vi "Configure Time Domain Reflection Type.vi"(7 "Cable Loss Value (0)":dbl, 8 "error in (no error)":errorcluster, 9 "Reflection Type (1: Round Trip)":i32(ring)=1 items=["One Way", "Round Trip"], 10 "Channel (1)":i32=1, 11 "VISA resource name":refnum<visa-resource-name>) -> (0 "error out":errorcluster, 3 "VISA resource name out":refnum<visa-resource-name>)   [LabVIEW 2011, in "Agilent ENA Series.lvlib"]
doc: "This VI configures time domain reflection type and cable loss value.\n\n<B>Note:</B>This VI is only vaild on E5061B."
uses:
  Agilent ENA Series.lvlib
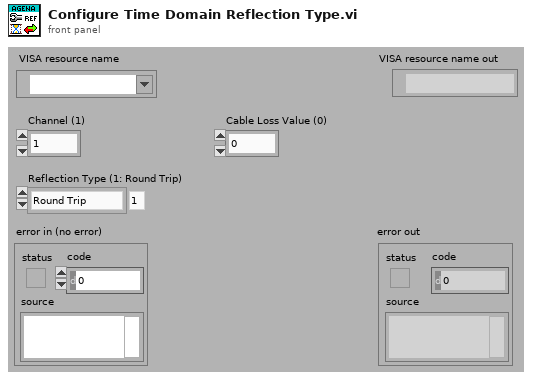
[diagram p1: front panel]
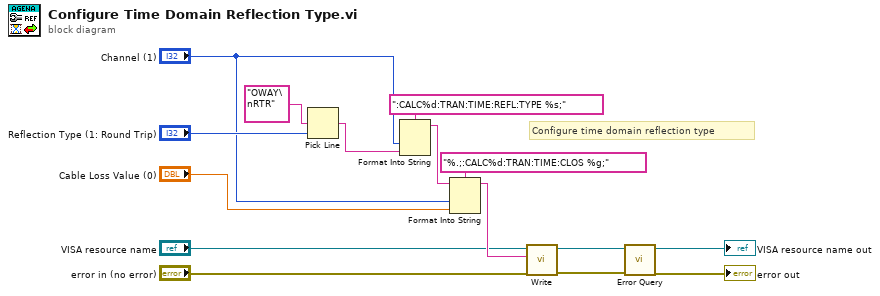
[diagram p0: block diagram]
diagram:
  # "Configure time domain reflection type"
  n1 = Pick Line(multi-line string="OWAY\nRTR", line index="Reflection Type (1: Round Trip)") -> (output string=w11:string)  [unwired: 1 out]
  n2 = Format Into String(format string=":CALC%d:TRAN:TIME:REFL:TYPE %s;", "Channel (1)", w11) -> (resulting string=w10:string)  [unwired: 2 in, 1 out]
  n3 = Format Into String(format string="%.;:CALC%d:TRAN:TIME:CLOS %g;", initial string=w10, "Channel (1)", "Cable Loss Value (0)") -> (resulting string=w5:string)  [unwired: 1 in, 1 out]
  n4 = call "Write.vi"("error in (no error)"="error in (no error)", "String ()"=w5, "VISA resource name"="VISA resource name") -> ("error out"=w1:errorcluster, "VISA resource name out"=w2:refnum<visa-resource-name>)  [unwired: 6 in, 1 out]
  n5 = call "Error Query.vi"("error in (no error)"=w1, "VISA resource name"=w2) -> ("error out"=→"error out":errorcluster, "VISA resource name out"=→"VISA resource name out":refnum<visa-resource-name>)  [unwired: 8 out]
